vi "Wash Needle Impl.vi"(8 "error in (no error)":errorcluster, 11 "Alltesta Autosampler in":refnum<class "Alltesta Autosampler.lvclass">) -> (0 "error out":errorcluster, 3 "Alltesta Autosampler out":refnum<class "Alltesta Autosampler.lvclass">)   [LabVIEW 2023, in "Alltesta Autosampler.lvlib" / "Alltesta Autosampler.lvclass"]
uses:
  Alltesta Autosampler.lvclass
  Alltesta Autosampler.lvclass/Alltesta Autosampler.ctl
  Alltesta Autosampler.lvlib
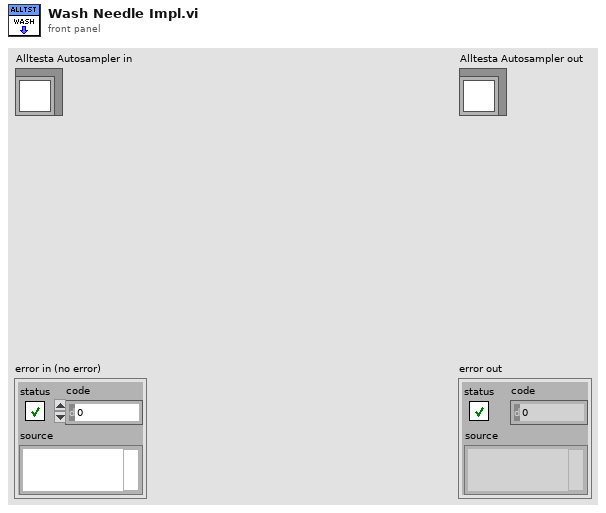
[diagram p1: front panel]
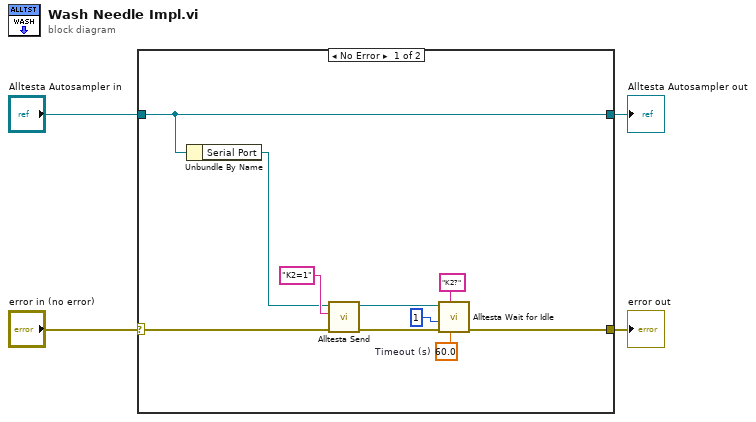
[diagram p0: block diagram]
diagram:
  n1 = case shown="No Error" "error in (no error)" {
    selector: "error in (no error)" -> [w12 w15]
    tunnel: [w9 w15] -> w3
    tunnel: "Alltesta Autosampler in" -> [w14 w16]
    tunnel: [w14 w16] -> w1
    frame No Error {
      w5 = 60.0  # Timeout (s)
      n2 = Unbundle By Name(w14) -> ("Serial Port"=w11:refnum<visa-resource-name>)
      n3 = call "Alltesta Send.vi"("error in (no error)"=w12, "Command"="K2=1" ("format string"), "Serial Port in"=w11) -> ("error out"=w10:errorcluster, "Serial Port out"=w8:refnum<visa-resource-name>)  [unwired: 6 in, 1 out]
      n4 = call "Alltesta Wait for Idle.vi"("Timeout (s)"=w5, "Poll Command"="K2?", "error in (no error)"=w10, "Lower Bound"=1, "Serial Port in"=w8) -> ("error out"=w9:errorcluster)  [unwired: 5 in, 1 out]
    }
    frame Error {
    }
  }
  "error out" <- w3
  "Alltesta Autosampler out" <- w1
